vi "poly_sub_filter_single_xwav.vi"(6 "add info? (T)":bool=TRUE, 8 "error in (no error)":errorcluster, 9 "f":i32=50 caption="base frequency (50Hz)", 10 "N":i32=3 caption="N of harmonics to remove (3)", 11 "xwave in":T1={"attributes"=variant, "X"={"start"=0.0, "delta"=0.0, "units"="index", "dim"="au"}, "Y"={"data"=[], "units"="au"}}) -> (0 "error out":errorcluster, 3 "xwave out":T1={"attributes"=variant, "X"={"start"=0.0, "delta"=0.0, "units"="index", "dim"="au"}, "Y"={"data"=[], "units"="au"}})   [LabVIEW 2015]
uses:
  xwave/xwav.ctl
  <vilib>/measure/matone.llb/Extract Single Tone Information 1 Chan.vi
  <vilib>/measure/NI_MAPro.lvlib
  <vilib>/Analysis/NI_AALBase.lvlib
panel:
  out "graph":cluster{dbl[], dbl[]}[](graph) caption="Automatic line filter level detection"
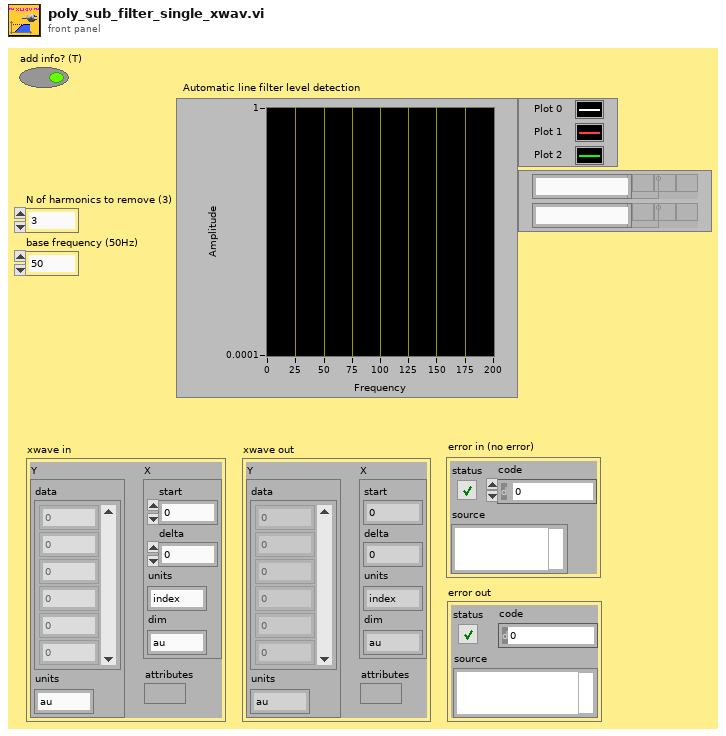
[diagram p1: front panel]
types:
  T1 = typedef "xwav.ctl" = cluster{"attributes":variant, "X":cluster{"start":dbl, "delta":dbl, "units":string, "dim":string}, "Y":cluster{"data":dbl[], "units":string}}
  T2 = enum32{"none", "input signal", "detected signal", "residual signal"}
  T3 = cluster{"approx freq. (optional)":dbl, "search (+/- % of Fsampl.)":dbl}
  T4 = cluster{"exported time signal":waveform(dbl), "exported spectrum (dB)":cluster{"f0":dbl, "df":dbl, "dB Spectrum (Hann)":dbl[]}}
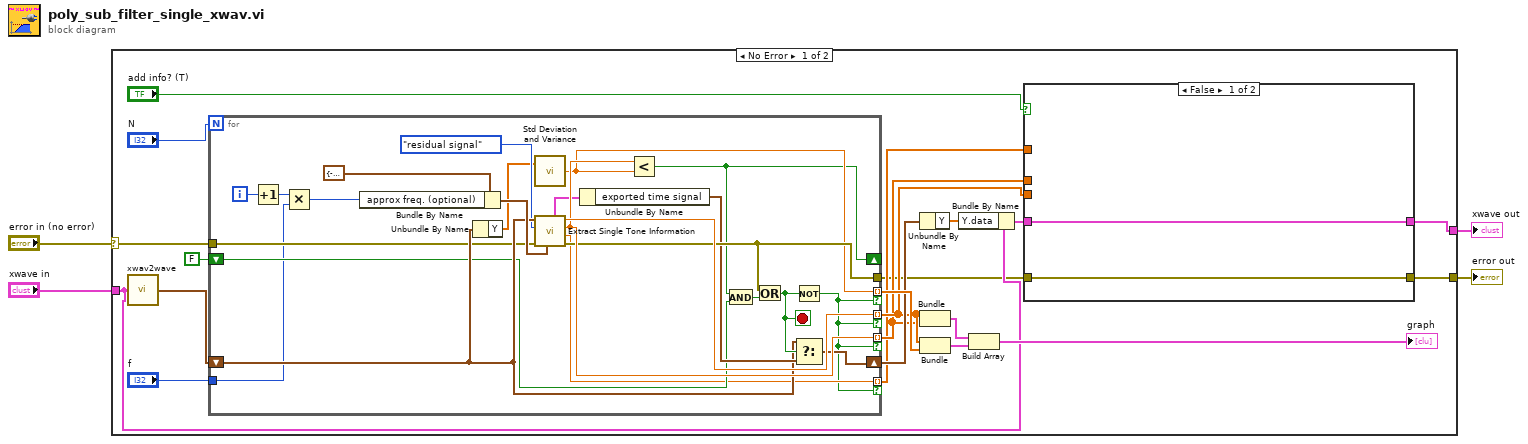
[diagram p0: block diagram]
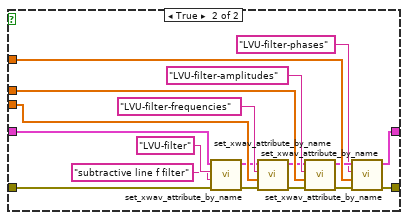
[diagram p2: hidden frame]
diagram:
  n1 = case shown="No Error" "error in (no error)" {
    selector: "error in (no error)" -> [w19 w68]
    tunnel: [w6 w68] -> w4
    tunnel: [w8 w69] -> w1
    tunnel: "xwave in" -> [w13 w69]
    frame No Error {
      n2 = call "xwav2wave.vi"("xwave"=w13) -> ("waveform"=w16:waveform(dbl))  [unwired: 4 in]
      n3 = for {
        N: "N" -> [_]
        shift-right: [w59] -> w15
        shift-left: w16 -> [w56]
        tunnel: [w67] -> w11 mode=indexing if=w48
        tunnel: [w60] -> w7
        tunnel: [w61] -> w10 mode=indexing if=w48
        tunnel: [w55] -> w23 mode=indexing if=w48
        shift-right: [w53] -> _
        shift-left: FALSE -> [w54]
        tunnel: w19 -> [w51]
        tunnel: "f" -> [w50]
        tunnel: [w49] -> w9 mode=indexing if=w48
        i -> [w64]
        stop <- w58 stop-if-true
        n4 = Increment(x=w64) -> (x+1=w63:i32)
        n5 = Multiply(x=w63, y=w50) -> (x*y=w62:i32)
        n6 = Bundle By Name(cluster=T3 {"approx freq. (optional)"=-1.0, "search (+/- % of Fsampl.)"=5.0} ("advanced search"), "approx freq. (optional)"=w62) -> (w65:T3)
        n7 = Unbundle By Name(w56) -> ("Y"=w46:dbl[])
        n8 = call <vilib>:"Std Deviation and Variance.vi"("X"=w46) -> ("standard deviation"=w55:dbl)  [unwired: 1 in, 2 out]
        n9 = call-poly <vilib>:"Extract Single Tone Information.vi"("advanced search"=w65, "error in (no error)"=w51, "export mode"=T2."residual signal", "time signal in"=w56) -> ("error out"=w60:errorcluster, "detected phase (deg)"=w49:dbl, "detected amplitude"=w61:dbl, "detected frequency"=w67:dbl, "exported signals"=w45:T4)  [unwired: 2 in, 1 out]
        n10 = Unbundle By Name(w45) -> ("exported time signal"=w57:waveform(dbl))
        n11 = Less?(x=w61, y=w55) -> (x < y?=w53:bool)
        n12 = And(x=w53, y=w54) -> (x .and. y?=w52:bool)
        n13 = Or(x=w60, y=w52) -> (x .or. y?=w58:bool)
        n14 = Not(x=w58) -> (.not. x?=w48:bool)
        n15 = Select(t=w56, s=w58, f=w57) -> (s? t:f=w59:waveform(dbl))
      }
      n16 = Unbundle By Name(w15) -> ("Y"=w14:dbl[])
      n17 = Bundle(w11, w10) -> (w22:cluster{dbl[], dbl[]})  [unwired: 1 in]
      n18 = Bundle(w11, w23) -> (w21:cluster{dbl[], dbl[]})  [unwired: 1 in]
      n19 = Bundle By Name(cluster=w13, "Y.data"=w14) -> (w12:T1)
      n20 = Build Array(w22, w21) -> (→"graph":cluster{dbl[], dbl[]}[])
      n21 = case shown="False" "add info? (T)" {
        tunnel: w12 -> [w26 w42]
        tunnel: w11 -> [_ w40]
        tunnel: w10 -> [_ w38]
        tunnel: w9 -> [_ w37]
        tunnel: [w26 w33] -> w8
        tunnel: w7 -> [w25 w32]
        tunnel: [w25 w28] -> w6
        frame False {
        }
        frame True {
          n22 = call "set_xwav_attribute_by_name.vi"("Error in"=w32, "value"="subtractive line f filter" ("name"), "name"="LVU-filter", "xwave in"=w42) -> ("Error out"=w31:errorcluster, "xwave out"=w36:T1)  [unwired: 5 in, 1 out]
          n23 = call "set_xwav_attribute_by_name.vi"("Error in"=w31, "value"=w40, "name"="LVU-filter-frequencies", "xwave in"=w36) -> ("Error out"=w30:errorcluster, "xwave out"=w35:T1)  [unwired: 5 in, 1 out]
          n24 = call "set_xwav_attribute_by_name.vi"("Error in"=w30, "value"=w38, "name"="LVU-filter-amplitudes", "xwave in"=w35) -> ("Error out"=w29:errorcluster, "xwave out"=w34:T1)  [unwired: 5 in, 1 out]
          n25 = call "set_xwav_attribute_by_name.vi"("Error in"=w29, "value"=w37, "name"="LVU-filter-phases", "xwave in"=w34) -> ("Error out"=w28:errorcluster, "xwave out"=w33:T1)  [unwired: 5 in, 1 out]
        }
      }
    }
    frame Error {
    }
  }
  "error out" <- w4
  "xwave out" <- w1
